vi "set_source_parameters_cluster.vi"(8 "error in (no error)":errorcluster, 9 "Source parameters":T1, 10 "Source number":u8, 11 "VISA resource name":refnum<visa-resource-name>) -> (0 "error out":errorcluster, 3 "VISA resource name out":refnum<visa-resource-name>)   [LabVIEW 2018]
doc: "Set the density of a material."
uses:
  Low Level/source_parameter_ring.ctl
  Low Level/source_parameters.ctl
panel:
  in  "Source parameter":T2 items=["DAC Output", "Shutter Output", "Number of Crucibles", "Crucible Output", "Turret Feedback", "Turret Input", "Turret Delay (s)"]
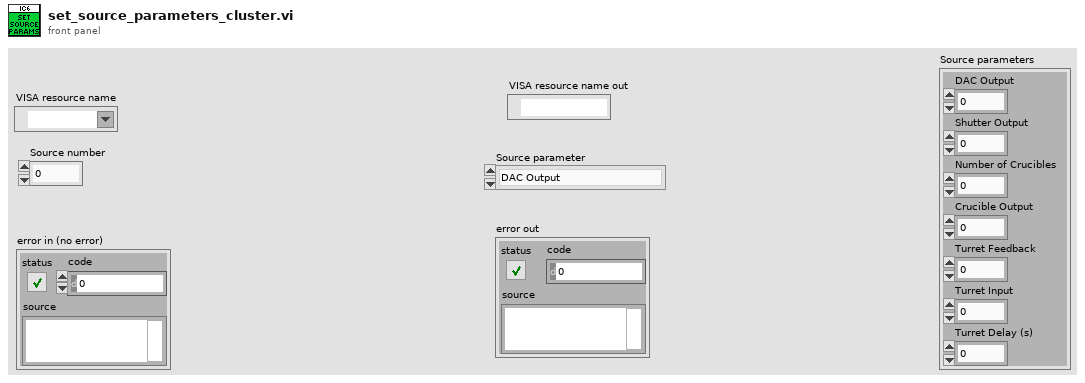
[diagram p1: front panel]
types:
  T1 = typedef "source_parameters.ctl" = cluster{"DAC Output":u8, "Shutter Output":u8, "Number of Crucibles":u8, "Crucible Output":u8, "Turret Feedback":u8, "Turret Input":u8, "Turret Delay (s)":u8}
  T2 = typedef "source_parameter_ring.ctl" = u16
  T3 = typedef "LVStringsAndValuesArrayTypeDef_U16.ctl" = cluster{"String":string, "Value":u16}[]
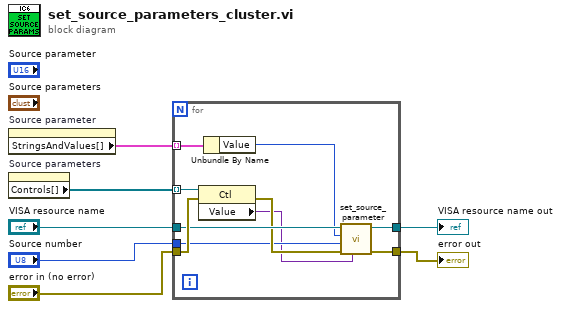
[diagram p0: block diagram]
diagram:
  n1 = property on="Source parameter" class="Ring (strict)"() -> ("StringsAndValues[]"=w3:T3)  [unwired: 2 in, 2 out]
  n2 = property on="Source parameters" class="Clust (strict)"() -> ("Controls[]"=w2:refnum<vi>[])  [unwired: 2 in, 2 out]
  n3 = for {
    tunnel: "VISA resource name" -> [w14]
    tunnel: [w13] -> w6
    tunnel: "error in (no error)" -> [w16]
    tunnel: "Source number" -> [w11]
    tunnel: w3 -> [w15] mode=indexing
    tunnel: w2 -> [w17] mode=indexing
    tunnel: [w8] -> w1
    n4 = property class="Ctl"(reference=w17, error in=w16) -> (error out=w12:errorcluster, "Value"=w10:variant)  [unwired: 1 out]
    n5 = Unbundle By Name(w15) -> ("Value"=w9:u16)
    n6 = call "set_source_parameter.vi"("Parameter"=w10, "error in (no error)"=w12, "Source number"=w11, "Source parameter"=w9, "VISA resource name"=w14) -> ("error out"=w8:errorcluster, "VISA resource name out"=w13:refnum<visa-resource-name>)  [unwired: 5 in]
  }
  "error out" <- w1
  "VISA resource name out" <- w6
